vi "2_1_VisualAD_Inference(Image).vi"() -> ()   [LabVIEW 2020]
uses:
  <vilib>/Ngene/DeepLTK Anomaly Detection Addon/Toolkit/API/Controls/NNPC_Setup.ctl
  <vilib>/Ngene/Deep Learning Toolkit/Toolkit/NN_Data/API/NN_Dims(C,H,W).ctl
  <vilib>/Ngene/Deep Learning Toolkit/Toolkit/NN_Network/Controls/NN_Device.ctl
  <vilib>/Ngene/DeepLTK Anomaly Detection Addon/Toolkit/API/Controls/Feature_Scorer_Params.ctl
  <vilib>/Ngene/DeepLTK Anomaly Detection Addon/Toolkit/API/Controls/Gaussian_Blur.ctl
  <vilib>/Ngene/DeepLTK Anomaly Detection Addon/Toolkit/API/Controls/NN_Paths.ctl
  subVIs/Visualizer/Controls/Display_Options.ctl
  subVIs/Visualizer/Controls/ROI_Display_Options.ctl
  subVIs/Visualizer/Controls/Heatmap_Display_Options.ctl
  subVIs/Visualizer/Controls/ColorMap.ctl
  <vilib>/Ngene/DeepLTK Anomaly Detection Addon/Toolkit/API/Controls/MinMax.ctl
  subVIs/Visualizer/Controls/Report_Images_CFG.ctl
  <vilib>/Ngene/DeepLTK Anomaly Detection Addon/Toolkit/API/NNPC_Predict/NNPC_Predict(Single).vi
  <vilib>/ptbypt/NI_PtbyPt.lvlib
  <vilib>/Ngene/DeepLTK Anomaly Detection Addon/Toolkit/DeepLTK_Anomaly_Detection_Addon.lvlib
  <vilib>/Ngene/Deep Learning Toolkit/Toolkit/Deep_Learning_Toolkit_by_Ngene.lvlib
panel:
  in  "Display_Options":T1={"ROI_Options"={"Color"=16860, "Width"=3, "Drawing Mode"=enum."Frame"}, "Heatmap_Options"={"ColorMap"=enum."Jet", "Alpha"=0.4, "Heatmap Range"={"Min"=25.0, "Max"=32.0}}, "Report_Images_CFG"={"Original Image"=TRUE, "Ground Truth"=FALSE, "HeatMap"=TRUE, "Mask"=TRUE, "Segmentation"=TRUE}} {"Heatmap_Options"."Heatmap Range"."Min" format="%#_5g"}
  out "dT_Init":dbl=1.6821560999960639 format="%#_3ps"
  in  "NNPC_Paths":T7={"CFG"=path "D:/Ngene/GitHub/deepltk_examples/3_Image_Processing/36_Anomaly_Detection/Models/NNPC_Cards_3ofHearts__25_10_21__19_21_13/NNPC_Cards_3ofHearts_25_10_21__19_21_13.cfg", "BIN"=path "D:/Ngene/GitHub/deepltk_examples/3_Image_Processing/36_Anomaly_Detection/Models/NNPC_Cards_3ofHearts__25_10_21__19_21_13/NNPC_Cards_3ofHearts_25_10_21__19_21_13.bin"}
  out "Image_Thrshld (Eval)":sgl=33.7813
  in  "Image_Thrshld(Custom)":sgl=-1.0 format="%_5g"
  out "dT_Predict":dbl=0.004892100999568356 format="%#_3ps"
  out "Pixel_Score(Min)":sgl=4.9043746
  out "Pixel_Score(Max)":sgl=34.97754
  out "Image_File_Path":path=path "D:/Ngene/GitHub/deepltk_examples/3_Image_Processing/36_Anomaly_Detection/Dataset/Playing_Cards_3ofHearts/test/bad/(219).png"
  in  "Feature_Scorer_Params":T8={"Nearest_Neighbors"=1, "Calculate Anomaly Map"=TRUE, "Gaussian_Blur"={"Kernel_Size"=33, "Sigma"=4.0}}
  out "Pixel_Thrshld (Eval)":sgl=26.7008
  in  "Stop":bool
  out "Anomaly?":bool=TRUE
  out "dT_ImRead":dbl=0.002781099989078939 format="%#_4ps"
  in  "NNPC_Setup":T10={"Input_Dims"={"C"=-1, "H"=-1, "W"=-1}, "mBatch"=1, "Device"=enum."GPU", "GPU Id"=0}
  out "Anomaly Detection Results":T13(plugin-control)
  out "Img_Score":sgl=38.33779
  in  "Image_idx":u32=39 max=49
  in  "Ground_Truth_Folder_Path":path
  in  "Pixel_Thrshld(Custom)":sgl=28.1 format="%_5g"
  in  "Test_Dataset_Folder_Path":path=path "D:/Ngene/GitHub/deepltk_examples/3_Image_Processing/36_Anomaly_Detection/Dataset/Playing_Cards_3ofHearts/test"
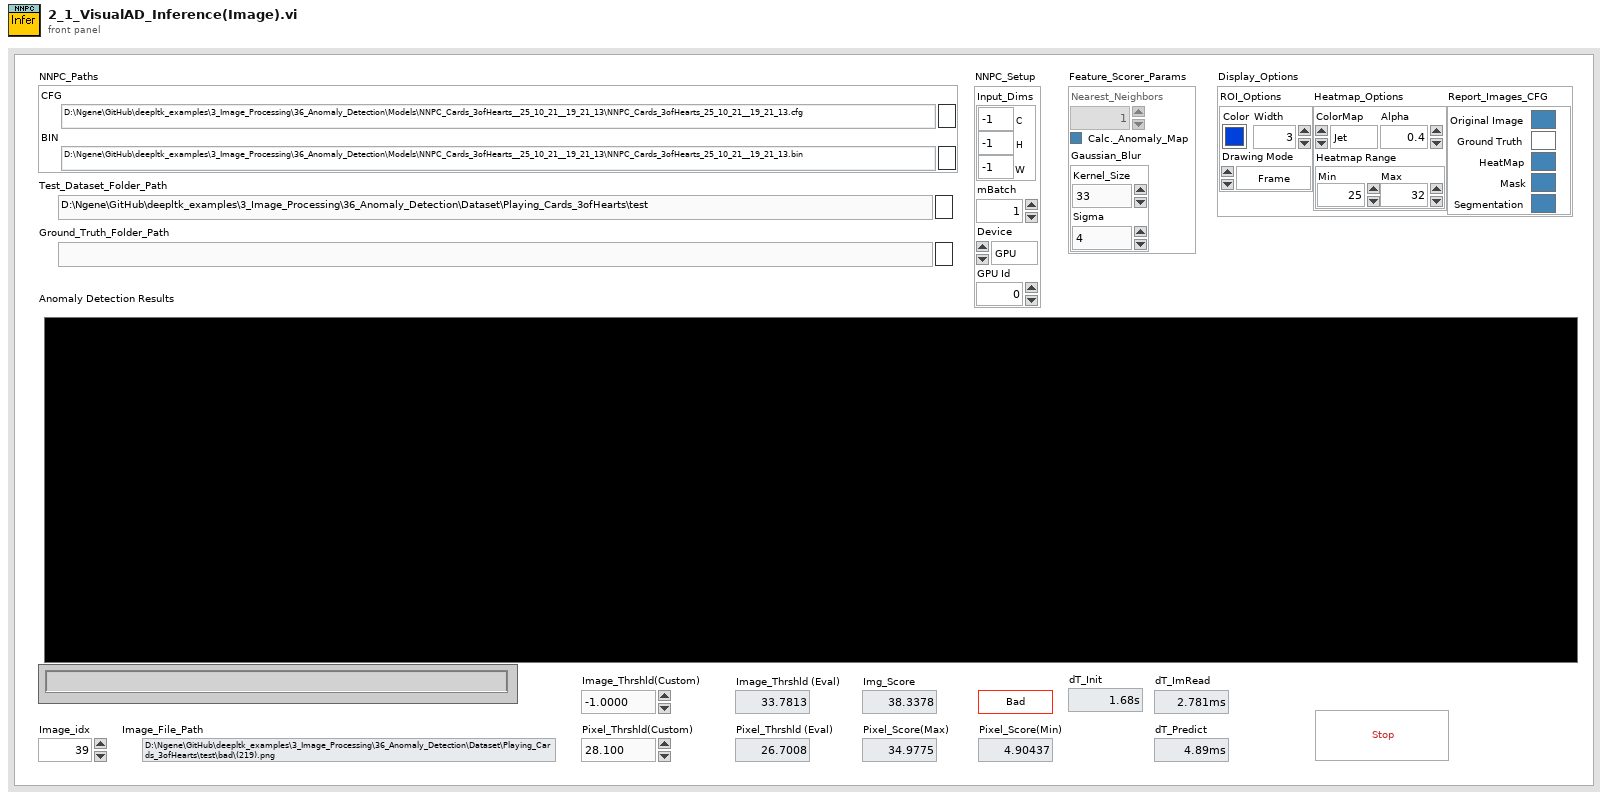
[diagram p1: front panel]
types:
  T1 = typedef "Display_Options.ctl" = cluster{"ROI_Options":T2, "Heatmap_Options":T3, "Report_Images_CFG":T6}
  T2 = typedef "ROI_Display_Options.ctl" = cluster{"Color":u32, "Width":u32, "Drawing Mode":enum16{"Frame", "Fill"}}
  T3 = typedef "Heatmap_Display_Options.ctl" = cluster{"ColorMap":T4, "Alpha":sgl, "Heatmap Range":T5}
  T4 = typedef "ColorMap.ctl" = enum16{"Jet", "Perula", "Inferno", "Plasma", "Viridis"}
  T5 = typedef "DeepLTK_Anomaly_Detection_Addon.lvlib/MinMax.ctl" = cluster{"Min":sgl, "Max":sgl}
  T6 = typedef "Report_Images_CFG.ctl" = cluster{"Original Image":bool, "Ground Truth":bool, "HeatMap":bool, "Mask":bool, "Segmentation":bool}
  T7 = typedef "DeepLTK_Anomaly_Detection_Addon.lvlib/NN_Paths.ctl" = cluster{"CFG":path, "BIN":path}
  T8 = typedef "DeepLTK_Anomaly_Detection_Addon.lvlib/Feature_Scorer_Params.ctl" = cluster{"Nearest_Neighbors":i32, "Calculate Anomaly Map":bool, "Gaussian_Blur":T9}
  T9 = typedef "DeepLTK_Anomaly_Detection_Addon.lvlib/Gaussian_Blur.ctl" = cluster{"Kernel_Size":i32, "Sigma":sgl}
  T10 = typedef "DeepLTK_Anomaly_Detection_Addon.lvlib/NNPC_Setup.ctl" = cluster{"Input_Dims":T11, "mBatch":i32, "Device":T12, "GPU Id":i32}
  T11 = typedef "Deep_Learning_Toolkit_by_Ngene.lvlib/NN_Dims(C,H,W).ctl" = cluster{"C":i32, "H":i32, "W":i32}
  T12 = typedef "Deep_Learning_Toolkit_by_Ngene.lvlib/NN_Device.ctl" = enum16{"CPU", "GPU"}
  T13 = typedef "IMAQ Image.ctl" = refnum<image>
  T14 = typedef "DeepLTK_Anomaly_Detection_Addon.lvlib/NNPC_Evaluation_Results.ctl" = cluster{"Threshold(Image)":sgl, "Threshold(Pixel)":sgl, "Pixel_Range":cluster{"Min":sgl, "Max":sgl}}
  T15 = typedef "DeepLTK_Anomaly_Detection_Addon.lvlib/NNPC_PreProcessing_Options.ctl" = cluster{"DS_Name":string, "Input_Dims":T11, "Cropping":T16, "Interpolation Type":u32, "MultiStage_ReSample?":bool, "Dataset_Stats":T17}
  T16 = typedef "DeepLTK_Anomaly_Detection_Addon.lvlib/Crop_CFG.ctl" = cluster{"Left":sgl, "Top":sgl, "Right":sgl, "Bottom":sgl}
  T17 = typedef "DeepLTK_Anomaly_Detection_Addon.lvlib/NNPC_DS_Stats.ctl" = cluster{"means":T18, "stds":T18}
  T18 = typedef "DeepLTK_Anomaly_Detection_Addon.lvlib/Image_Stats_RGB.ctl" = cluster{"R":sgl, "G":sgl, "B":sgl}
  T19 = typedef "DeepLTK_Anomaly_Detection_Addon.lvlib/NNPC_Instance.ctl" = cluster{"Name":string, "NN":T20, "MemBank_Data":T34}
  T20 = typedef "Deep_Learning_Toolkit_by_Ngene.lvlib/NN.ctl" = cluster{"Name":string, "No of Layers":i32, "mBatch":i32, "Layers":T21[], "Dimty":T22, "Dims_In":T11, "Dims_Out":T11, "Working_Dir":path, "Train?":bool, "Train_Params":T23, "LR_Update_Policy":T26, "Session Data":T28, "Ground_truth":T29, "NNg_hdls":T30, "NN_Device":T12, "GPU Id":i32, "Labels":string[], "Loss_Type":T31, "Loss_Cfg_Prms":variant, "NNG_WS":T32, "DryRun?":bool}
  T21 = typedef "Deep_Learning_Toolkit_by_Ngene.lvlib/NN_Layer_ref.ctl" = refnum<file>
  T22 = typedef "Deep_Learning_Toolkit_by_Ngene.lvlib/NN_In_Out_Dim-ty.ctl" = enum8{"In1D_Out1D", "In3D_Out1D", "In3D_Out3D", "In3D_OutBBox"}
  T23 = typedef "Deep_Learning_Toolkit_by_Ngene.lvlib/NN_Train_Params.ctl" = cluster{"Optimizer":T24, "Beta_1":sgl, "Beta_2":sgl, "Weight Decay(L1)":sgl, "Weight Decay(L2)":sgl, "Data_Sampling":T25}
  T24 = typedef "Deep_Learning_Toolkit_by_Ngene.lvlib/NN_Train_Optimizer.ctl" = enum16{"SGD", "Adam", "Adagrad", "Adadelta", "RMSProp", "Nesterov"}
  T25 = typedef "Deep_Learning_Toolkit_by_Ngene.lvlib/NN_Train_Data_Sampling.ctl" = enum16{"Random", "Sequential"}
  T26 = typedef "Deep_Learning_Toolkit_by_Ngene.lvlib/NN_LR_Policy_Cfg.ctl" = cluster{"Policy_Type":T27, "LR0":dbl, "k":sgl, "WarmUp_Policy":enum16{"Step", "Ramp"}, "WarmUp_Iter":i32, "WarmUp_Ratio":sgl}
  T27 = typedef "Deep_Learning_Toolkit_by_Ngene.lvlib/NN_LR_Policy_Type.ctl" = enum16{"Manual", "Step", "Exp", "1/t"}
  T28 = typedef "Deep_Learning_Toolkit_by_Ngene.lvlib/NN_Train_Session_Data.ctl" = cluster{"Epochs":sgl, "Tot_Iter":i32, "LR":sgl, "LR_iter":i32}
  T29 = typedef "Deep_Learning_Toolkit_by_Ngene.lvlib/NN_Ground_truth.ctl" = cluster{"Y":variant}
  T30 = typedef "Deep_Learning_Toolkit_by_Ngene.lvlib/nng_cuda_handles.ctl" = cluster{"cudnn":u64, "cublas":u64, "stream":u64, "curand":u64}
  T31 = typedef "Deep_Learning_Toolkit_by_Ngene.lvlib/NN_Loss_Type.ctl" = enum16{"None", "MSE", "CrossEntropy", "YOLO_v2", "YOLO_v4"}
  T32 = typedef "Deep_Learning_Toolkit_by_Ngene.lvlib/NNG_WS.ctl" = cluster{"NNG_WS_Mem":T33, "Max_WS_Size":i64}
  T33 = typedef "Deep_Learning_Toolkit_by_Ngene.lvlib/NNg_WS_Mem_DVR.ctl" = refnum<data-value>
  T34 = typedef "DeepLTK_Anomaly_Detection_Addon.lvlib/MemBank_and_Norm_Variants.ctl" = cluster{"MemBank":variant, "MemBank Norm":variant}
  T35 = typedef "Anomaly_Detection_Results_Imgs.ctl" = cluster{"Image":T13, "Ground Truth":T13, "Predicted Heat Map":T13, "Predicted Mask":T13, "Segmentation":T13}
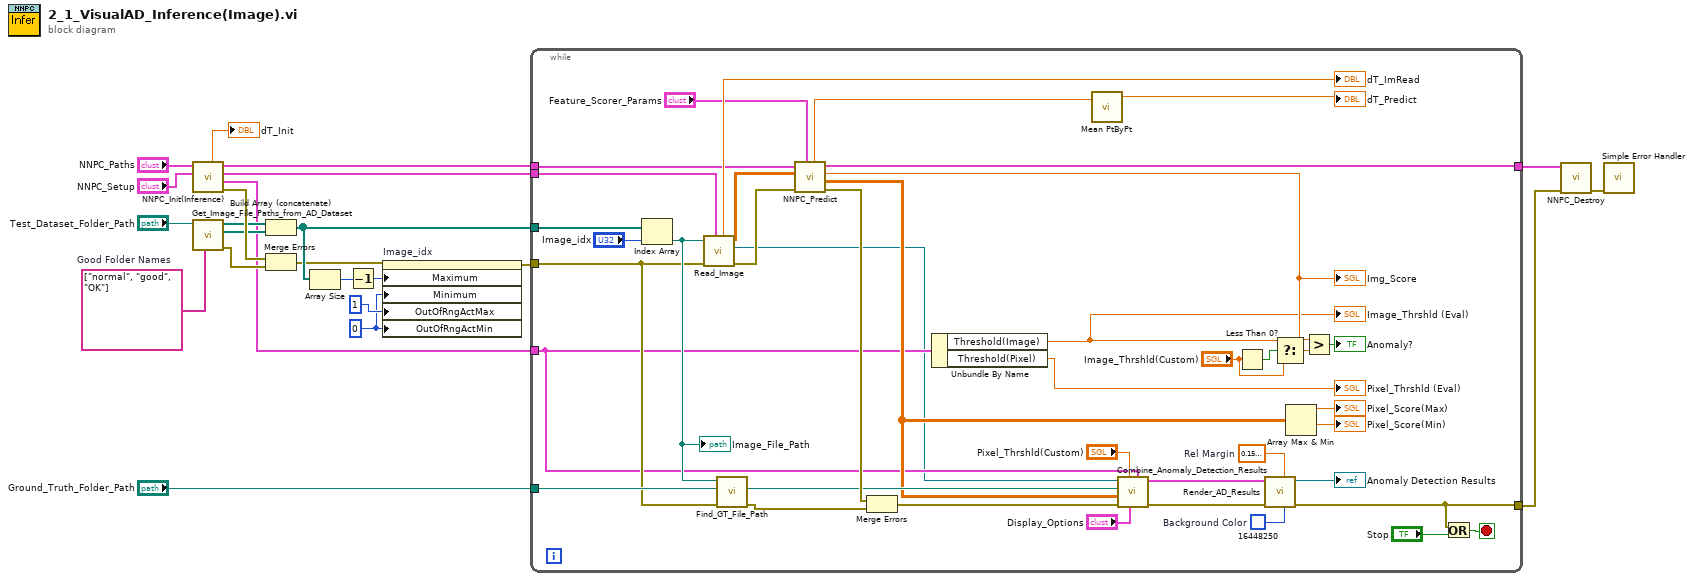
[diagram p0: block diagram]
diagram:
  w1 = string[] ["normal", "good", "OK"]  # Good Folder Names
  w3 = u32 0 ("Data Entry Limits:Minimum")
  n1 = call <vilib>:"NNPC_Init(Inference).vi"("NNPC_Setup"="NNPC_Setup", "NNPC_Paths"="NNPC_Paths") -> ("error out"=w21:errorcluster, "Evaluation_Results"=w4:T14, "PreProc_Options"=w6:T15, "NNPC_out"=w22:T19, "dT_Init_Inference"=→"dT_Init":dbl)  [unwired: 5 in]
  n2 = call "Get_Image_File_Paths_from_AD_Dataset.vi"("Good Folder Names"=w1, "Dataset Folder"="Test_Dataset_Folder_Path") -> ("error out"=w18:errorcluster, "Bad Dataset Files"=w14:path[], "Good Dataset Files"=w13:path[])  [unwired: 7 in]
  n3 = Build Array (concatenate)(w13, w14) -> (w19:path[])
  n4 = Merge Errors(w21, w18) -> (w8:errorcluster)
  n5 = Array Size(array=w19) -> (size(s)=w9:i32)
  n6 = Decrement(x=w9) -> (x-1=w11:i32)
  n7 = property on="Image_idx" class="DigNum (strict)"(error in=w8, "Maximum"=w11, "Minimum"=w3, "OutOfRngActMax"=u8 1 ("Response to Value Outside Limits:Maximum"), "OutOfRngActMin"=w3) -> (error out=w7:errorcluster)  [unwired: 1 in, 1 out]
  n8 = while {
    tunnel: w19 -> [w63]
    tunnel: w22 -> [w46]
    tunnel: [w40] -> w16
    tunnel: w7 -> [w36]
    tunnel: [w37] -> w17
    tunnel: "Ground_Truth_Folder_Path" -> [w49]
    tunnel: w6 -> [w33]
    tunnel: w4 -> [w29]
    stop <- w38 stop-if-true
    w25 = u32 16448250  # Background Color
    w26 = sgl 0.15  # Rel Margin
    n9 = Index Array(array=w63, index="Image_idx") -> (element=w51:path)
    "Image_File_Path" <- w51
    n10 = call "Read_Image.vi"("PreProcessing_Options"=w33, "error in"=w36, "Img Path"=w51) -> ("error out"=w41:errorcluster, 2:"Image Out (Preproc)"=w28:T13, 3:"Image Out (Preproc)"=w27:sgl[][][], "dT_Img_Read"=→"dT_ImRead":dbl)  [unwired: 3 in, 2 out]
    n11 = call "Find_GT_File_Path.vi"("error in"=w36, "GT Mask Folder Path"=w49, "Image File Path"=w51) -> ("error out"=w34:errorcluster, "GT File Path"=w50:path)  [unwired: 5 in, 2 out]
    n12 = call-poly <vilib>:"NNPC_Predict.vi"("Feature_Scorer_Params"="Feature_Scorer_Params", "error in"=w41, "Image_in"=w27, "NNPC_in"=w46) -> ("error out"=w61:errorcluster, "Anomaly_Map"=w45:sgl[][], "Pred_Score"=w44:sgl, "NNPC_out"=w40:T19, "dT_Predict"=w32:dbl)  [unwired: 2 in, 1 out]
    "Img_Score" <- w44
    n13 = Merge Errors(w61, w34) -> (w35:errorcluster)
    n14 = Unbundle By Name(w29) -> ("Threshold(Image)"=w31:sgl, "Threshold(Pixel)"=→"Pixel_Thrshld (Eval)":sgl)
    "Image_Thrshld (Eval)" <- w31
    n15 = call <vilib>:"Mean PtByPt.vi"("x"=w32) -> ("mean"=→"dT_Predict":dbl)  [unwired: 3 in, 1 out]
    n16 = call "Combine_Anomaly_Detection_Results.vi"("Evaluation_Results"=w29, "Display_Options"="Display_Options", "Pixel Anomaly Thrshld"="Pixel_Thrshld(Custom)", "error in"=w35, "Anomaly Map"=w45, "Gt File Path"=w50, "Orig Image In"=w28) -> ("error out"=w60:errorcluster, "Anomaly Detection Results"=w59:T35)  [unwired: 2 in, 1 out]
    n17 = Less Than 0?(x="Image_Thrshld(Custom)") -> (x < 0?=w55:bool)
    n18 = call "Render_AD_Results.vi"("Background Color"=w25, "Rel._Margin"=w26, "error in"=w60, "Anomaly Detection Rresults"=w59) -> ("error out"=w37:errorcluster, "Anomaly Detection Results"=→"Anomaly Detection Results":T13)  [unwired: 6 in]
    n19 = Select(t=w31, s=w55, f="Image_Thrshld(Custom)") -> (s? t:f=w53:sgl)
    n20 = Array Max & Min(array=w45) -> (max value=→"Pixel_Score(Max)":sgl, min value=→"Pixel_Score(Min)":sgl)  [unwired: 2 out]
    n21 = Greater?(x=w44, y=w53) -> (0:→"Anomaly?":bool)
    n22 = Or(x=w37, y="Stop") -> (x .or. y?=w38:bool)
  }
  n23 = call <vilib>:"NNPC_Destroy.vi"("error in"=w17, "NNPC_in"=w16) -> ("error out"=w15:errorcluster)  [unwired: 9 in]
  n24 = call <vilib>:"Simple Error Handler.vi"("error in (no error)"=w15) -> ()  [unwired: 4 in, 5 out]
